vi "Periodic Tasks.vi"(8 "error in":errorcluster) -> ()   [LabVIEW 2016]
doc: "This VI runs in parallel to other tasks. It can contain as many user-defined periodic loops as you need. These can carry out PID or other sorts of timed response."
uses:
  Typedefs/typedef_enum_Joystick Axes.ctl
  Typedefs/typedef_enum_Start Position.ctl
  <vilib>/Rock Robotics/SystemInterfaces/Utilities/FPGA_UtilitiesLED Source.ctl
  <vilib>/Rock Robotics/SystemInterfaces/Utilities/FPGA_UtilitiesLED State.ctl
  Typedefs/typedef_enum_Defense.ctl
  <vilib>/Rock Robotics/WPI/Utilities/WPI_GetSetVariantRefNum.vi
  Robot Global Data.vi
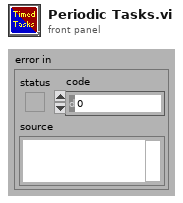
[diagram p1: front panel]
types:
  T1 = typedef "WPI_JoystickDevRef.ctl" = cluster{"Device":T2}
  T2 = typedef "WPI_JoystickDeviceEnum.ctl" = enum16{"USB 0", "USB 1", "USB 2", "USB 3", "USB 4", "USB 5"}
  T3 = typedef "typedef_enum_Joystick Axes.ctl" = enum16{"LeftRight", "ForeBack", "Twist", "Throttle"}
  T4 = typedef "typedef_enum_Defense.ctl" = enum16{"Low Bar", "A) Portcullis", "A) Cheval de Frise", "B) Moat", "B) Ramparts", "C) Drawbridge", "C) Sally Port", "D) Rock Wall", "D) Rough Terrain"}
  T5 = typedef "typedef_enum_Start Position.ctl" = enum16{"1", "2", "3", "4", "5"}
  T6 = typedef "FPGA_UtilitiesLED State.ctl" = enum16{"Off", "On", "Toggle"}
  T7 = typedef "FPGA_UtilitiesLED Source.ctl" = enum16{"User LED", "FPGA LED"}
  T8 = typedef "WPI_CompressorDevRef.ctl" = cluster{"DevStatus":errorcluster, "Pneumatics Control Module":u8}
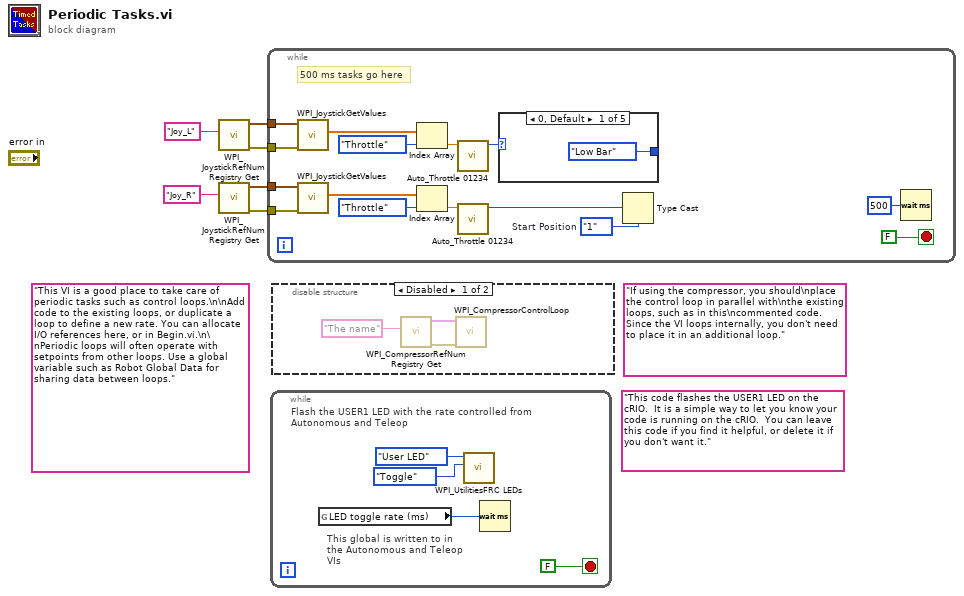
[diagram p0: block diagram]
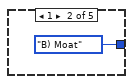
[diagram p3: hidden frame]
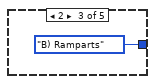
[diagram p4: hidden frame]
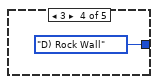
[diagram p5: hidden frame]
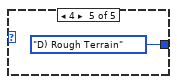
[diagram p6: hidden frame]
diagram:
  (unwired) "If using the compressor, you should\nplace the control loop in parallel with\nthe existing loops, such as in this\ncommented code. Since the VI loops internally, you don't need to place it in an additional loop."
  (unwired) "This code flashes the USER1 LED on the cRIO.  It is a simple way to let you know your code is running on the cRIO.  You can leave this code if you find it helpful, or delete it if you don't want it."
  (unwired) "This VI is a good place to take care of periodic tasks such as control loops.\n\nAdd code to the existing loops, or duplicate a loop to define a new rate. You can allocate I/O references here, or in Begin.vi.\n\nPeriodic loops will often operate with setpoints from other loops. Use a global variable such as Robot Global Data for sharing data between loops."
  n1 = call <vilib>:"WPI_JoystickRefNum Registry Get.vi"("refnum name"="Joy_L") -> ("error out"=w1:errorcluster, "JoystickDevRef"=w4:T1)  [unwired: 1 in, 8 out]
  n2 = call <vilib>:"WPI_JoystickRefNum Registry Get.vi"("refnum name"="Joy_R") -> ("error out"=w2:errorcluster, "JoystickDevRef"=w3:T1)  [unwired: 1 in, 8 out]
  n3 = while {
    tunnel: w4 -> [w10]
    tunnel: w3 -> [w9]
    tunnel: w2 -> [w8]
    tunnel: w1 -> [w7]
    stop <- FALSE stop-if-true
    w19 = typedef_enum_Start_Position."1"  # Start Position
    # "500 ms tasks go here"
    n4 = call <vilib>:"WPI_JoystickGetValues.vi"("error in (no error)"=w7, "JoystickDevRef"=w10) -> ("Axes"=w12:dbl[])  [unwired: 5 in, 4 out]
    n5 = call <vilib>:"WPI_JoystickGetValues.vi"("error in (no error)"=w8, "JoystickDevRef"=w9) -> ("Axes"=w13:dbl[])  [unwired: 5 in, 4 out]
    n6 = Index Array(array=w12, index=typedef_enum_Joystick_Axes."Throttle") -> (element=w15:dbl)
    n7 = Index Array(array=w13, index=typedef_enum_Joystick_Axes."Throttle") -> (element=w16:dbl)
    n8 = call "Auto_Throttle 01234.vi"("Throttle"=w15) -> ("01234"=w17:u16)  [unwired: 10 in]
    n9 = call "Auto_Throttle 01234.vi"("Throttle"=w16) -> ("01234"=w18:u16)  [unwired: 10 in]
    n10 = case shown="0, Default" w17 {
      tunnel: [typedef_enum_Defense."Low Bar" ("Defense") typedef_enum_Defense."B) Moat" ("Defense") typedef_enum_Defense."B) Ramparts" ("Defense") typedef_enum_Defense."D) Rock Wall" ("Defense") typedef_enum_Defense."D) Rough Terrain" ("Defense")] -> _
      frame 0, Default {
      }
      frame 1 {
      }
      frame 2 {
      }
      frame 3 {
      }
      frame 4 {
      }
    }
    n11 = Type Cast(type=w19, x=w18) -> ()  [unwired: 1 out]
    n12 = Wait (ms)(milliseconds to wait=u32 500) -> ()  [unwired: 1 out]
  }
  n13 = while {
    stop <- FALSE stop-if-true
    # "This global is written to in the Autonomous and Teleop VIs"
    # "Flash the USER1 LED with the rate controlled from Autonomous and Teleop"
    n14 = global read "Robot Global Data.vi" "LED toggle rate (ms)"() -> (w27:u32)
    n15 = call <vilib>:"WPI_UtilitiesFRC LEDs.vi"("State"=FPGA_UtilitiesLED_State."Toggle", "LED Type"=FPGA_UtilitiesLED_Source."User LED") -> ()  [unwired: 1 in, 9 out]
    n16 = Wait (ms)(milliseconds to wait=w27) -> ()  [unwired: 1 out]
  }
  n17 = disable-structure shown="Disabled" {
    frame Disabled {
      n18 = call <vilib>:"WPI_CompressorRefNum Registry Get.vi"("refnum name"="The name") -> ("error out"=w31:errorcluster, "CompressorDevRef"=w33:T8)  [unwired: 9 in]
      n19 = call <vilib>:"WPI_CompressorControlLoop.vi"("error in (no error)"=w31, "CompressorDevRef"=w33) -> ()  [unwired: 10 in]
    }
    frame Enabled {
    }
  }
